vi "Read Session.vi"(8 "error in (no error)":errorcluster, 11 "UnitTestFramework in":refnum<class "UnitTestFramework.lvclass">) -> (0 "error out":errorcluster, 2 "Session":i32, 3 "UnitTestFramework out":refnum<class "UnitTestFramework.lvclass">)   [LabVIEW 2019, in "UnitTestFramework.lvclass"]
uses:
  UnitTestFramework.lvclass
  UnitTestFramework.lvclass/UnitTestFramework.ctl
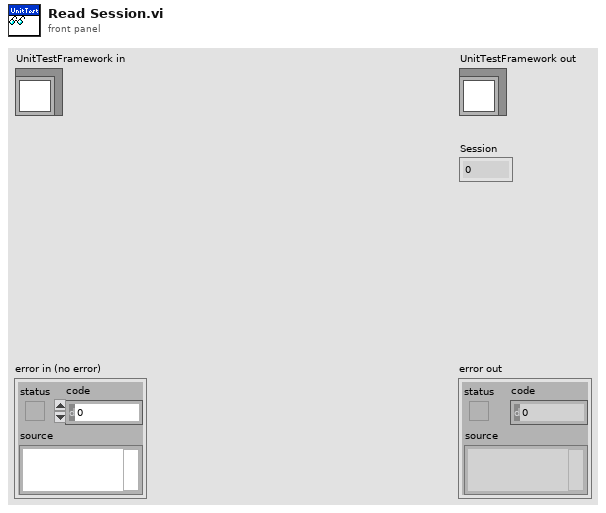
[diagram p1: front panel]
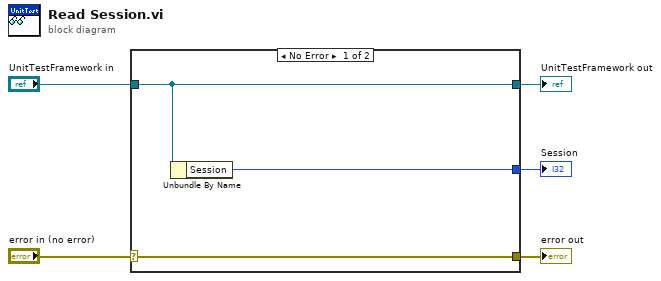
[diagram p0: block diagram]
diagram:
  n1 = case shown="No Error" "error in (no error)" {
    selector: "error in (no error)" -> [w8 w9]
    tunnel: [w8 w9] -> w4
    tunnel: [w7 w10] -> w2
    tunnel: "UnitTestFramework in" -> [w7 w10]
    tunnel: [w6 _] -> w1
    frame No Error {
      n2 = Unbundle By Name(w7) -> ("Session"=w6:i32)
    }
    frame Error {
    }
  }
  "error out" <- w4
  "UnitTestFramework out" <- w2
  "Session" <- w1
